vi "Seq Dialog Check LVDT's Position.vi"(9 "Segment Data":T2={"Name"="Check LVDT's", "Description"="", "data string"="\u0000\u0000\u0000\u0007\u0000\u0000\u0000\u0002?ð\u0000\u0000\u0000\u0000\u0000\u0000¿ð\u0000\u0000\u0000\u0000\u0000\u0000?ð\u0000\u0000\u0000\u0000\u0000\u0000¿ð\u0000\u0000\u0000\u0000\u0000\u0000?ð\u0000\u0000\u0000\u0000\u0000\u0000¿ð\u0000\u0000\u0000\u0000\u0000\u0000?ð\u0000\u0000\u0000\u0000\u0000\u0000¿ð\u0000\u0000\u0000\u0000\u0000\u0000?ð\u0000\u0000\u0000\u0000\u0000\u0000¿ð\u0000\u0000\u0000\u0000\u0000\u0000?ð\u0000\u0000\u0000\u0000\u0000\u0000¿ð\u0000\u0000\u0000\u0000\u0000\u0000?ð\u0000\u0000\u0000\u0000\u0000\u0000¿ð\u0000\u0000\u0000\u0000\u0000\u0000"}) -> (0 "Step Hisitory":string[](array[string]), 1 "Segment Data 2":T2)   [LabVIEW 2018]
uses:
  type defs/Sequence Info.ctl
  type defs/EOL LVDT's Check Controller.ctl
  type defs/config paths for seq def.ctl
  <vilib>/Utility/config.llb/Read Key (String).vi
  <vilib>/Utility/config.llb/NI_LVConfig.lvlib
panel:
  in  "LVDT's Limit Array":T1[](array[typedef])=[{"Upper Limit"=100.0, "Lower Limit"=-100.0, "LVDT Name"="LVDT 1", "Check"=TRUE}, {"Upper Limit"=100.0, "Lower Limit"=-100.0, "LVDT Name"="LVDT 2", "Check"=TRUE}, {"Upper Limit"=100.0, "Lower Limit"=-100.0, "LVDT Name"="LVDT 3", "Check"=TRUE}, {"Upper Limit"=100.0, "Lower Limit"=-100.0, "LVDT Name"="LVDT 4", "Check"=TRUE}, {"Upper Limit"=100.0, "Lower Limit"=-100.0, "LVDT Name"="LVDT 5", "Check"=TRUE}, {"Upper Limit"=100.0, "Lower Limit"=-100.0, "LVDT Name"="LVDT 6", "Check"=TRUE}, {"Upper Limit"=100.0, "Lower Limit"=-100.0, "LVDT Name"="LVDT 7", "Check"=TRUE}, {"Upper Limit"=100.0, "Lower Limit"=-100.0, "LVDT Name"="LVDT 8", "Check"=TRUE}, {"Upper Limit"=100.0, "Lower Limit"=-100.0, "LVDT Name"="LVDT 9", "Check"=TRUE}, {"Upper Limit"=100.0, "Lower Limit"=-100.0, "LVDT Name"="LVDT 10", "Check"=TRUE}, {"Upper Limit"=100.0, "Lower Limit"=-100.0, "LVDT Name"="LVDT 11", "Check"=TRUE}, {"Upper Limit"=100.0, "Lower Limit"=-100.0, "LVDT Name"="LVDT 12", "Check"=TRUE}, {"Upper Limit"=100.0, "Lower Limit"=-100.0, "LVDT Name"="LVDT 13", "Check"=TRUE}, {"Upper Limit"=100.0, "Lower Limit"=-100.0, "LVDT Name"="LVDT 14", "Check"=TRUE}, {"Upper Limit"=100.0, "Lower Limit"=-100.0, "LVDT Name"="LVDT 15", "Check"=TRUE}] {"Lower Limit" format="%.2f"; "Upper Limit" format="%.2f"}
  out "Name":string="Audit Check LVDT's"
  in  "Description":string
  in  "Save":bool
  in  "Cancel":bool
  # "LVDT Name"
  # "Upper Limit"
  # "Lower Limit"
  # "Check"
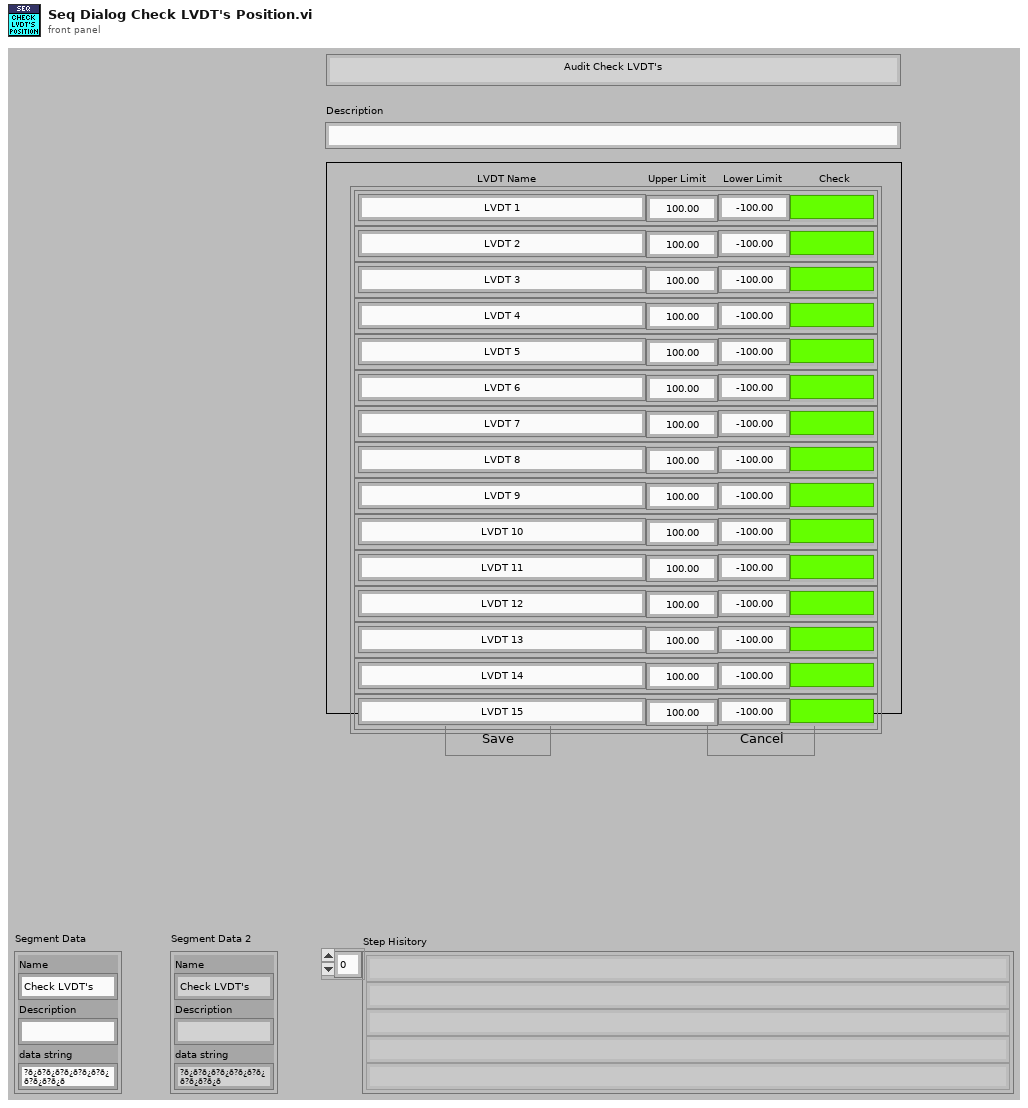
[diagram p1: front panel]
types:
  T1 = typedef "EOL LVDT's Check Controller.ctl" = cluster{"Upper Limit":dbl, "Lower Limit":dbl, "LVDT Name":string, "Check":bool}
  T2 = typedef "Sequence Info.ctl" = cluster{"Name":string, "Description":string, "data string":string}
  T3 = typedef "config paths for seq def.ctl" = cluster{"Part Type":string, "base path":path}
  T4 = cluster{"LVDT's Limit Array":T1[], "Segment Data":T2, "Old Data":string, "New Data":string, "config paths":T3}
  T5 = typedef "NI_LVConfig.lvlib/Config Data RefNum.ctl" = refnum<k1>
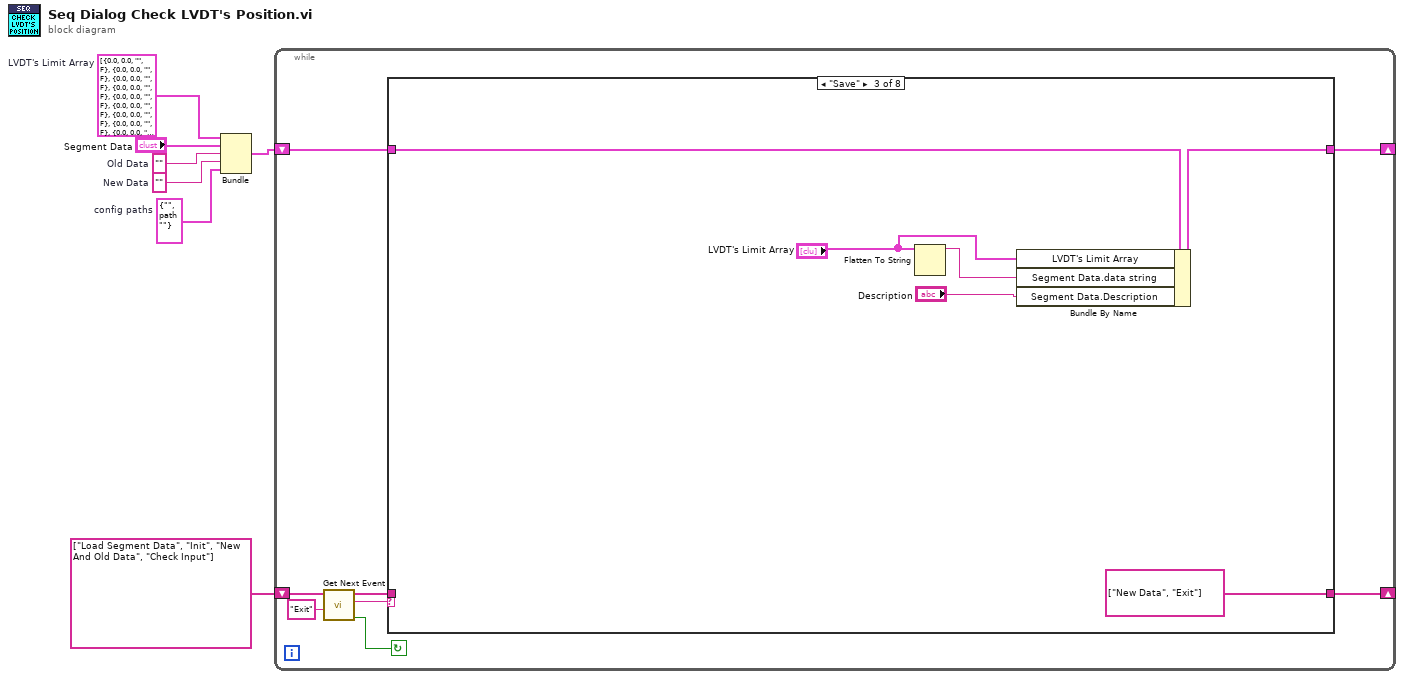
[diagram p0: block diagram]
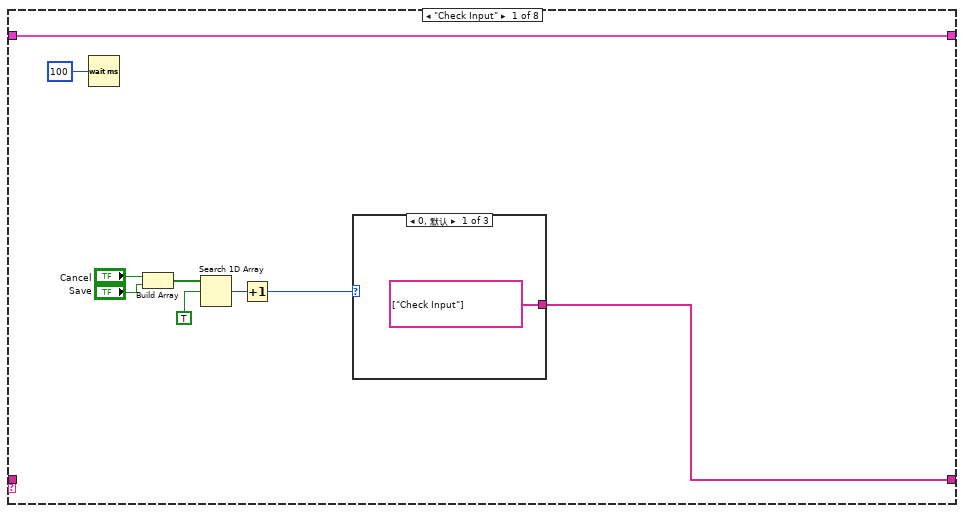
[diagram p2: hidden frame]
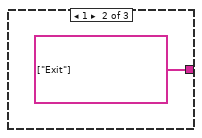
[diagram p3: hidden frame]
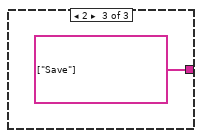
[diagram p4: hidden frame]
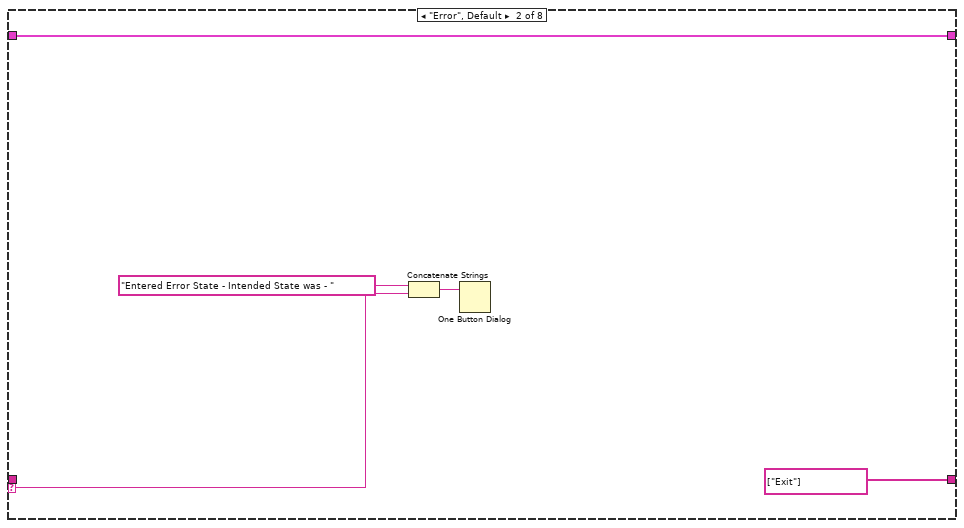
[diagram p5: hidden frame]
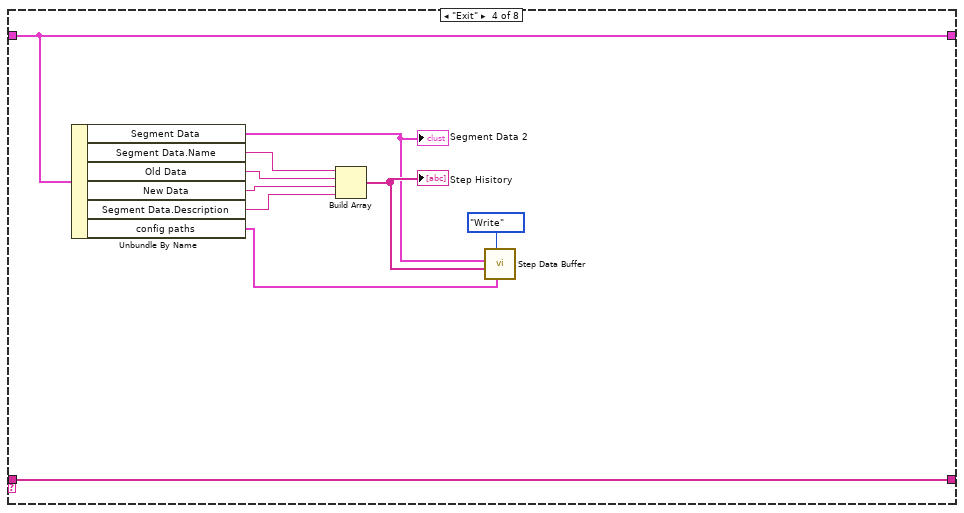
[diagram p6: hidden frame]
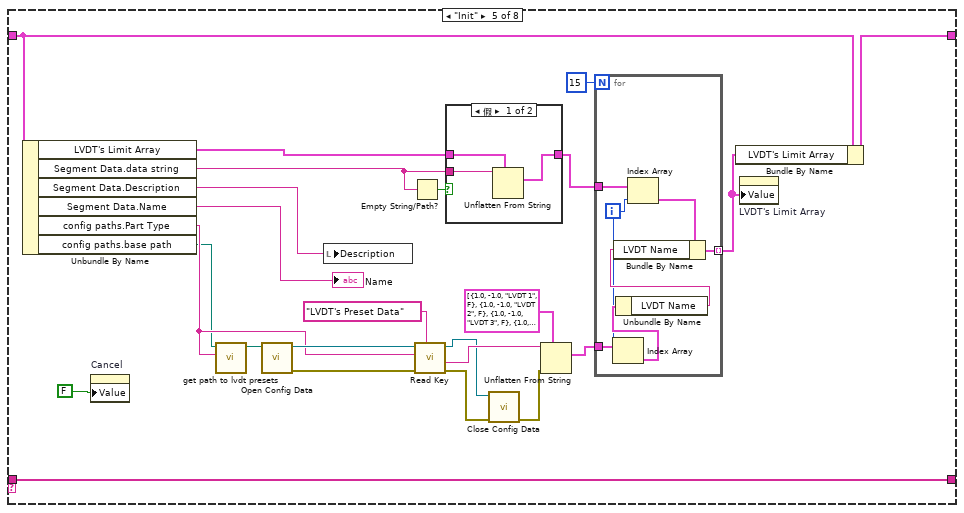
[diagram p7: hidden frame]
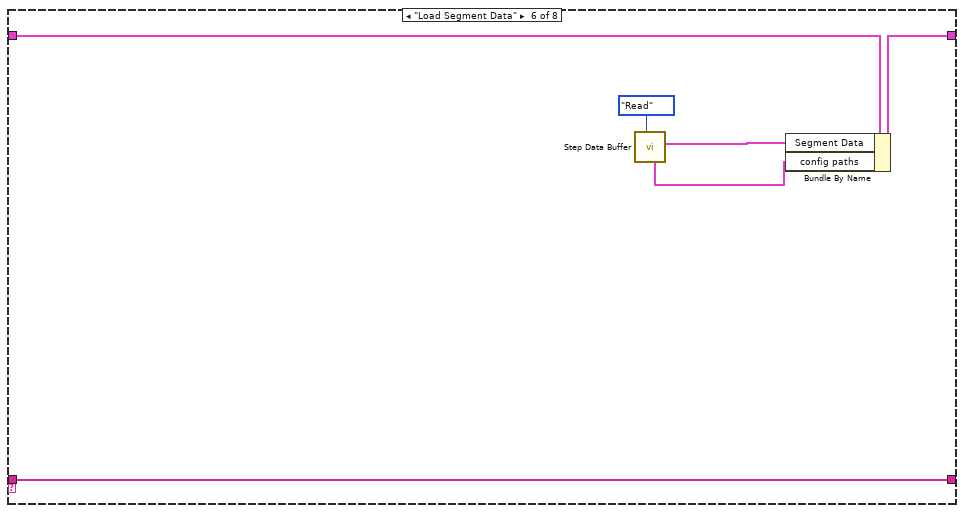
[diagram p9: hidden frame]
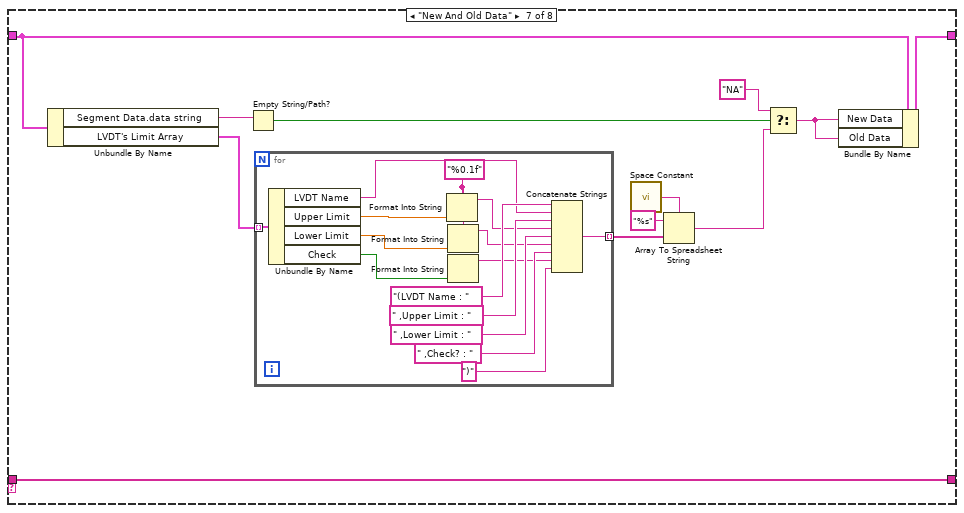
[diagram p10: hidden frame]
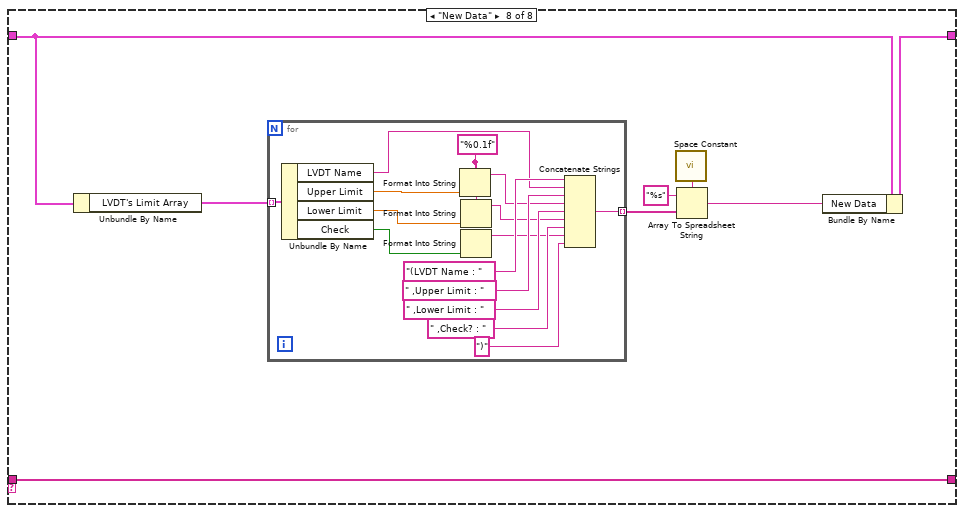
[diagram p11: hidden frame]
diagram:
  w1 = T3 {"Part Type"="", "base path"=path ""}  # config paths
  w2 = T1[] [{"Upper Limit"=0.0, "Lower Limit"=0.0, "LVDT Name"="", "Check"=FALSE}, {"Upper Limit"=0.0, "Lower Limit"=0.0, "LVDT Name"="", "Check"=FALSE}, {"Upper Limit"=0.0, "Lower Limit"=0.0, "LVDT Name"="", "Check"=FALSE}, {"Upper Limit"=0.0, "Lower Limit"=0.0, "LVDT Name"="", "Check"=FALSE}, {"Upper Limit"=0.0, "Lower Limit"=0.0, "LVDT Name"="", "Check"=FALSE}, {"Upper Limit"=0.0, "Lower Limit"=0.0, "LVDT Name"="", "Check"=FALSE}, {"Upper Limit"=0.0, "Lower Limit"=0.0, "LVDT Name"="", "Check"=FALSE}, {"Upper Limit"=0.0, "Lower Limit"=0.0, "LVDT Name"="", "Check"=FALSE}, {"Upper Limit"=0.0, "Lower Limit"=0.0, "LVDT Name"="", "Check"=FALSE}, {"Upper Limit"=0.0, "Lower Limit"=0.0, "LVDT Name"="", "Check"=FALSE}, {"Upper Limit"=0.0, "Lower Limit"=0.0, "LVDT Name"="", "Check"=FALSE}, {"Upper Limit"=0.0, "Lower Limit"=0.0, "LVDT Name"="", "Check"=FALSE}]  # LVDT's Limit Array
  w4 = ""  # New Data
  w5 = ""  # Old Data
  n1 = Bundle("LVDT's Limit Array"=w2, "Segment Data"="Segment Data", "Old Data"=w5, "New Data"=w4, "config paths"=w1) -> (w7:T4)  [unwired: 1 in]
  n2 = while {
    shift-right: [w13] -> _
    shift-left: string[] ["Load Segment Data", "Init", "New And Old Data", "Check Input"] ("Event queue out") -> [w12]
    shift-right: [w8] -> _
    shift-left: w7 -> [w9]
    stop <- w11 continue-if-true
    n3 = call "Get Next Event.vi"("Exit Event"="Exit", "event queue in"=w12) -> ("Condition (Exit:F)"=w11:bool, "next event"=w15:string, "event queue out"=w14:string[])  [unwired: 3 in]
    n4 = case shown="\"Save\"" w15 {
      selector: w15 -> [_ w29 _ _ _ _ _ _]
      tunnel: w14 -> [_ _ _ w48 w72 w89 w101 w124]
      tunnel: [w18 string[] ["Exit"] ("event queue out") string[] ["New Data", "Exit"] ("Event queue out") w48 w72 w89 w101 w124] -> w13
      tunnel: w9 -> [w23 w28 w38 w44 w67 w86 w96 w123]
      tunnel: [w23 w28 w37 w44 w66 w85 w95 w122] -> w8
      frame "Check Input" {
        n5 = Wait (ms)(milliseconds to wait=u32 100) -> ()  [unwired: 1 out]
        n6 = Build Array("Cancel", "Save") -> (w20:bool[])
        n7 = Search 1D Array(1D array=w20, element=TRUE) -> (index of element=w21:i32)  [unwired: 1 in]
        n8 = Increment(x=w21) -> (x+1=w22:i32)
        n9 = case shown="0, 默认" w22 {
          tunnel: [string[] ["Check Input"] ("Events to Insert") string[] ["Exit"] ("Events to Insert") string[] ["Save"] ("Events to Insert")] -> w18
          frame 0, Default {
          }
          frame 1 {
          }
          frame 2 {
          }
        }
      }
      frame "Error", Default {
        n10 = Concatenate Strings("Entered Error State - Intended State was - " ("string"), w29) -> (w32:string)
        n11 = One Button Dialog(message=w32) -> ()  [unwired: 1 in, 1 out]
      }
      frame "Save" {
        n12 = Flatten To String(anything="LVDT's Limit Array") -> (data string=w35:string)  [unwired: 3 in, 2 out]
        n13 = Bundle By Name(cluster=w38, "LVDT's Limit Array"="LVDT's Limit Array", "Segment Data.data string"=w35, "Segment Data.Description"="Description") -> (w37:T4)
      }
      frame "Exit" {
        n14 = Unbundle By Name(w44) -> ("Segment Data"=w41:T2, "Segment Data.Name"=w46:string, "Old Data"=w45:string, "New Data"=w47:string, "Segment Data.Description"=w40:string, "config paths"=w39:T3)
        "Segment Data 2" <- w41
        n15 = Build Array(w46, w45, w47, w40) -> (w42:string[])
        "Step Hisitory" <- w42
        n16 = call "Step Data Buffer.vi"("config paths"=w39, "Mode"=enum16{"Init", "Read", "Write"}."Write", "Step Hisitory In"=w42, "Segment Data In"=w41) -> ()  [unwired: 3 in, 5 out]
      }
      frame "Init" {
        n17 = Unbundle By Name(w67) -> ("LVDT's Limit Array"=w71:T1[], "Segment Data.data string"=w70:string, "Segment Data.Description"=w68:string, "Segment Data.Name"=→"Name":string, "config paths.Part Type"=w51:string, "config paths.base path"=w49:path)
        n18 = property on="Cancel" class="Bool (严格)"("Value"=FALSE ("Cancel")) -> ()  [unwired: 2 in, 2 out]
        n19 = call "get path to lvdt presets.vi"("product"=w51, "paths.Base Path"=w49) -> ("path"=w56:path)  [unwired: 9 in]
        n20 = call <vilib>:"Open Config Data.vi"("configuration file path"=w56) -> ("error out"=w59:errorcluster, "refnum"=w60:T5)  [unwired: 8 in, 1 out]
        n21 = local write "Description"(w68) -> ()
        n22 = Empty String/Path?(string/path=w70) -> (empty?=w69:bool)
        n23 = call-poly <vilib>:"Read Key.vi"("section"="LVDT's Preset Data", "error in (no error)"=w59, "key"=w51, "refnum"=w60) -> ("error out"=w55:errorcluster, "value"=w57:string, "refnum out"=w53:T5)  [unwired: 4 in, 1 out]
        n24 = case shown="假" w69 {
          tunnel: w71 -> [w82 w83]
          tunnel: w70 -> [w81 _]
          tunnel: [w80 w83] -> w63
          frame False {
            n25 = Unflatten From String(type=w82, binary string=w81) -> (value=w80:T1[])  [unwired: 3 in, 2 out]
          }
          frame True {
          }
        }
        n26 = call <vilib>:"Close Config Data.vi"("error in (no error)"=w55, "refnum"=w53) -> ("error out"=w54:errorcluster)  [unwired: 8 in, 1 out]
        n27 = Unflatten From String(type=T1[] [{"Upper Limit"=1.0, "Lower Limit"=-1.0, "LVDT Name"="LVDT 1", "Check"=FALSE}, {"Upper Limit"=1.0, "Lower Limit"=-1.0, "LVDT Name"="LVDT 2", "Check"=FALSE}, {"Upper Limit"=1.0, "Lower Limit"=-1.0, "LVDT Name"="LVDT 3", "Check"=FALSE}, {"Upper Limit"=1.0, "Lower Limit"=-1.0, "LVDT Name"="LVDT 4", "Check"=FALSE}, {"Upper Limit"=1.0, "Lower Limit"=-1.0, "LVDT Name"="LVDT 5", "Check"=FALSE}, {"Upper Limit"=1.0, "Lower Limit"=-1.0, "LVDT Name"="LVDT 6", "Check"=FALSE}, {"Upper Limit"=1.0, "Lower Limit"=-1.0, "LVDT Name"="LVDT 7", "Check"=FALSE}, {"Upper Limit"=1.0, "Lower Limit"=-1.0, "LVDT Name"="LVDT 8", "Check"=FALSE}, {"Upper Limit"=1.0, "Lower Limit"=-1.0, "LVDT Name"="LVDT 9", "Check"=FALSE}, {"Upper Limit"=1.0, "Lower Limit"=-1.0, "LVDT Name"="LVDT 10", "Check"=FALSE}, {"Upper Limit"=1.0, "Lower Limit"=-1.0, "LVDT Name"="LVDT 11", "Check"=FALSE}, {"Upper Limit"=1.0, "Lower Limit"=-1.0, "LVDT Name"="LVDT 12", "Check"=FALSE}, {"Upper Limit"=1.0, "Lower Limit"=-1.0, "LVDT Name"="LVDT 13", "Check"=FALSE}, {"Upper Limit"=1.0, "Lower Limit"=-1.0, "LVDT Name"="LVDT 14", "Check"=FALSE}] ("WK LVDT's Limit Array"), binary string=w57, error in (no error)=w54) -> (value=w52:T1[])  [unwired: 2 in, 2 out]
        n28 = for {
          N: 15 -> [_]
          tunnel: w63 -> [w79]
          tunnel: [w77] -> w62 mode=indexing
          tunnel: w52 -> [w76]
          i -> [w73]
          n29 = Index Array(array=w76, index=w73) -> (element=w74:T1)
          n30 = Unbundle By Name(w74) -> ("LVDT Name"=w75:string)
          n31 = Index Array(array=w79, index=w73) -> (element=w78:T1)
          n32 = Bundle By Name(cluster=w78, "LVDT Name"=w75) -> (w77:T1)
        }
        n33 = Bundle By Name(cluster=w67, "LVDT's Limit Array"=w62) -> (w66:T4)
        n34 = property on="LVDT's Limit Array" class="Arr (严格)"("Value"=w62) -> ()  [unwired: 2 in, 2 out]
      }
      frame "Load Segment Data" {
        n35 = call "Step Data Buffer.vi"("Mode"=enum16{"Init", "Read", "Write"}."Read") -> ("Segment Data Out"=w88:T2, "config paths"=w84:T3)  [unwired: 6 in, 3 out]
        n36 = Bundle By Name(cluster=w86, "Segment Data"=w88, "config paths"=w84) -> (w85:T4)
      }
      frame "New And Old Data" {
        n37 = Unbundle By Name(w96) -> ("Segment Data.data string"=w100:string, "LVDT's Limit Array"=w94:T1[])
        n38 = Empty String/Path?(string/path=w100) -> (empty?=w99:bool)
        n39 = for {
          tunnel: w94 -> [w114] mode=indexing
          tunnel: [w104] -> w93 mode=indexing
          w103 = "%0.1f" ("format string")
          n40 = Unbundle By Name(w114) -> ("LVDT Name"=w108:string, "Upper Limit"=w111:dbl, "Lower Limit"=w110:dbl, "Check"=w109:bool)
          n41 = Format Into String(format string=w103, w111) -> (resulting string=w107:string)  [unwired: 2 in, 1 out]
          n42 = Format Into String(format string=w103, w110) -> (resulting string=w106:string)  [unwired: 2 in, 1 out]
          n43 = Format Into String(w109) -> (resulting string=w105:string)  [unwired: 3 in, 1 out]
          n44 = Concatenate Strings("(LVDT Name : " ("string"), w108, " ,Upper Limit : " ("string"), w107, " ,Lower Limit : " ("string"), w106, " ,Check? : " ("string"), w105, ")" ("string")) -> (w104:string)
        }
        n45 = call <vilib>:"Space Constant.vi"() -> ("String"=w90:string)
        n46 = Array To Spreadsheet String(delimiter (Tab)=w90, array=w93, 3:"%s" ("format string")) -> (spreadsheet string=w92:string)
        n47 = Select(t="NA", s=w99, f=w92) -> (s? t:f=w97:string)
        n48 = Bundle By Name(cluster=w96, "New Data"=w97, "Old Data"=w97) -> (w95:T4)
      }
      frame "New Data" {
        n49 = Unbundle By Name(w123) -> ("LVDT's Limit Array"=w118:T1[])
        n50 = for {
          tunnel: w118 -> [w137] mode=indexing
          tunnel: [w127] -> w121 mode=indexing
          w126 = "%0.1f" ("format string")
          n51 = Unbundle By Name(w137) -> ("LVDT Name"=w131:string, "Upper Limit"=w134:dbl, "Lower Limit"=w133:dbl, "Check"=w132:bool)
          n52 = Format Into String(format string=w126, w134) -> (resulting string=w130:string)  [unwired: 2 in, 1 out]
          n53 = Format Into String(format string=w126, w133) -> (resulting string=w129:string)  [unwired: 2 in, 1 out]
          n54 = Format Into String(w132) -> (resulting string=w128:string)  [unwired: 3 in, 1 out]
          n55 = Concatenate Strings("(LVDT Name : " ("string"), w131, " ,Upper Limit : " ("string"), w130, " ,Lower Limit : " ("string"), w129, " ,Check? : " ("string"), w128, ")" ("string")) -> (w127:string)
        }
        n56 = call <vilib>:"Space Constant.vi"() -> ("String"=w119:string)
        n57 = Array To Spreadsheet String(delimiter (Tab)=w119, array=w121, 3:"%s" ("format string")) -> (spreadsheet string=w117:string)
        n58 = Bundle By Name(cluster=w123, "New Data"=w117) -> (w122:T4)
      }
    }
  }
